vi "process.vi"(8 "error in (no error)":errorcluster, 10 "input":sgl[][](array[numeric]), 11 "DL090629NoiseTraceProcessor in":refnum<class "TraceProcessorDL090629Noise.lvclass">) -> (0 "error out":errorcluster, 2 "output":sgl[][](array[numeric]), 3 "DL090629NoiseTraceProcessor out":refnum<class "TraceProcessorDL090629Noise.lvclass">)   [LabVIEW 2010, in "TraceProcessorDL090629Noise.lvclass"]
uses:
  TraceProcessorDL090629Noise.lvclass
  <vilib>/Analysis/NI_AALBase.lvlib
panel:
  out "standard deviations":dbl[](graph)
  in  "sampling window":i32=10 min=1
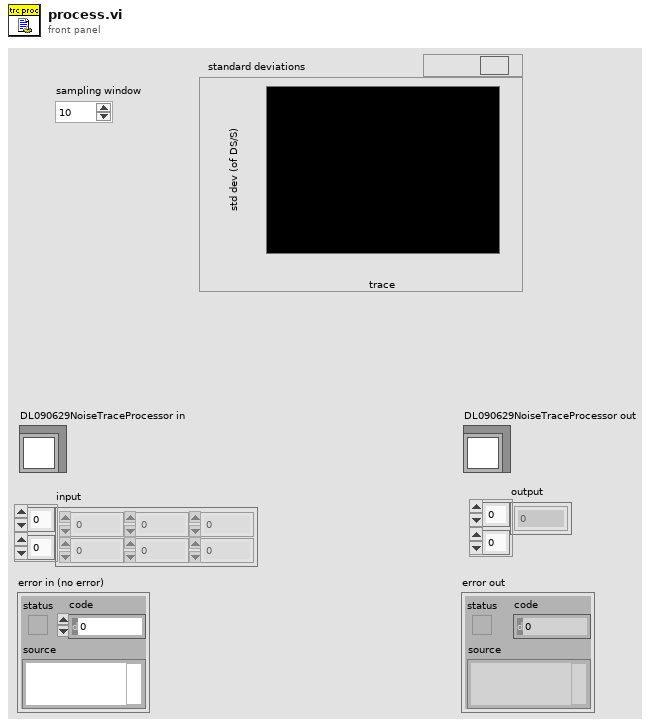
[diagram p1: front panel]
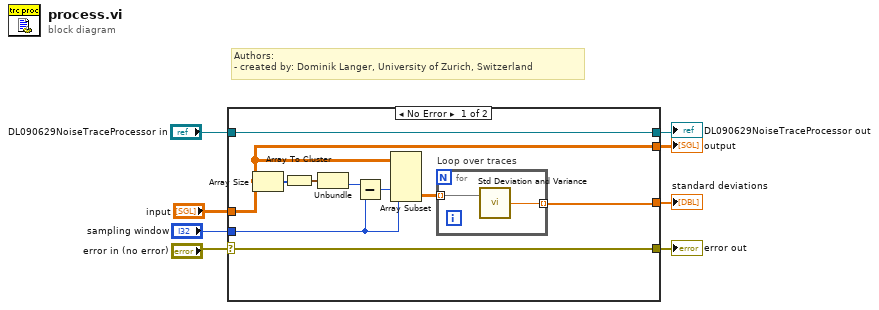
[diagram p0: block diagram]
diagram:
  # "Authors: \n- created by: Dominik Langer, University of Zurich, Switzerland"
  n1 = case shown="No Error" "error in (no error)" {
    selector: "error in (no error)" -> [w18 w21]
    tunnel: "DL090629NoiseTraceProcessor in" -> [w17 w22]
    tunnel: [w18 w21] -> w6
    tunnel: [w17 w22] -> w5
    tunnel: [w11 w23] -> w3
    tunnel: "input" -> [w11 w23]
    tunnel: "sampling window" -> [w14 _]
    tunnel: [w9 _] -> w1
    frame No Error {
      n2 = Array Size(array=w11) -> (size(s)=w16:i32[])
      n3 = Array To Cluster(array=w16) -> (cluster=w15:cluster{"[0]":i32, "[1]":i32})
      n4 = Unbundle(w15) -> ("[1]"=w12:i32)  [unwired: 1 out]
      n5 = Subtract(x=w12, y=w14) -> (x-y=w13:i32)
      n6 = Array Subset(array=w11, index (col)=w13, length (col)=w14) -> (w10:sgl[][])  [unwired: 2 in]
      n7 = for "Loop over traces" {
        tunnel: w10 -> [w20] mode=indexing
        tunnel: [w19] -> w9 mode=indexing
        n8 = call <vilib>:"Std Deviation and Variance.vi"("X"=w20) -> ("standard deviation"=w19:dbl)  [unwired: 1 in, 2 out]
      }
    }
    frame Error {
    }
  }
  "error out" <- w6
  "DL090629NoiseTraceProcessor out" <- w5
  "output" <- w3
  "standard deviations" <- w1
